vi "PID Advanced (DBL Array) Obsolete.vi"(0 "setpoint":dbl[](array[numeric])=[0.0] format="%.2f", 1 "output range":cluster{"output high":dbl, "output low":dbl}[](array[cluster])=[{"output high"=100.0, "output low"=-100.0}] {"output low" format="%.2f"; "output high" format="%.2f"}, 2 "auto? (T)":bool[](array[boolean])=[TRUE], 3 "manual control":dbl[](array[numeric])=[0.0] format="%.2f", 5 "process variable":dbl[](array[numeric])=[0.0] format="%.2f", 7 "setpoint range":T2(array[cluster])=[{"setpoint high"=100.0, "setpoint low"=0.0}] {"setpoint high" format="%.2f"; "setpoint low" format="%.2f"}, 9 "PID gains":T1(array[cluster])=[{"proportional gain (Kc)"=1.0, "integral time (Ti, min)"=0.01, "derivative time (Td, min)"=0.0}] {"derivative time (Td, min)" format="%.3f"; "integral time (Ti, min)" format="%.3f"; "proportional gain (Kc)" format="%.3f"}, 11 "dt (s)":dbl=-1.0 format="%.3f", 12 "reinitialize? (F)":bool, 13 "beta":dbl[](array[numeric])=[1.0] format="%.2f", 14 "linearity":dbl[](array[numeric])=[1.0] format="%.2f") -> (4 "output":dbl[](array[numeric]) format="%.2f", 15 "dt out (s)":dbl format="%.3f")   [LabVIEW 2017, in "NI_PID_pid.lvlib"]
doc: "PID algorithm with advanced optional features. PID algorithm includes features of PID.vi as well as manual mode control with bumpless manual to automatic transitions, non-linear integral action, two degree of freedom control and error-squared control."
uses:
  <vilib>/addons/control/pid/NI_PID_pid.lvlib
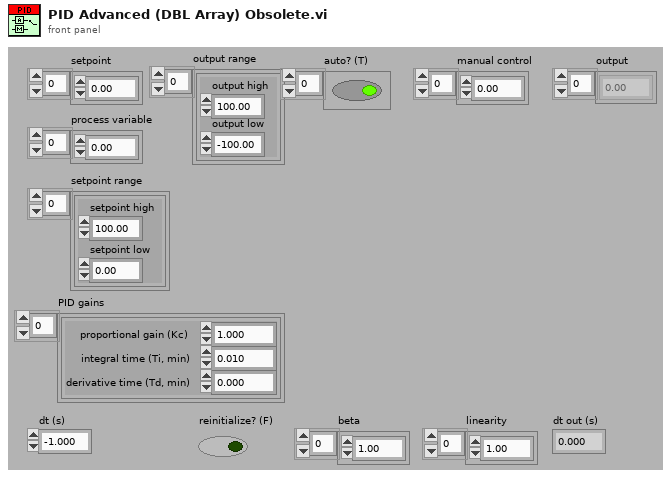
[diagram p1: front panel]
types:
  T1 = cluster{"proportional gain (Kc)":dbl, "integral time (Ti, min)":dbl, "derivative time (Td, min)":dbl}[]
  T2 = cluster{"setpoint high":dbl, "setpoint low":dbl}[]
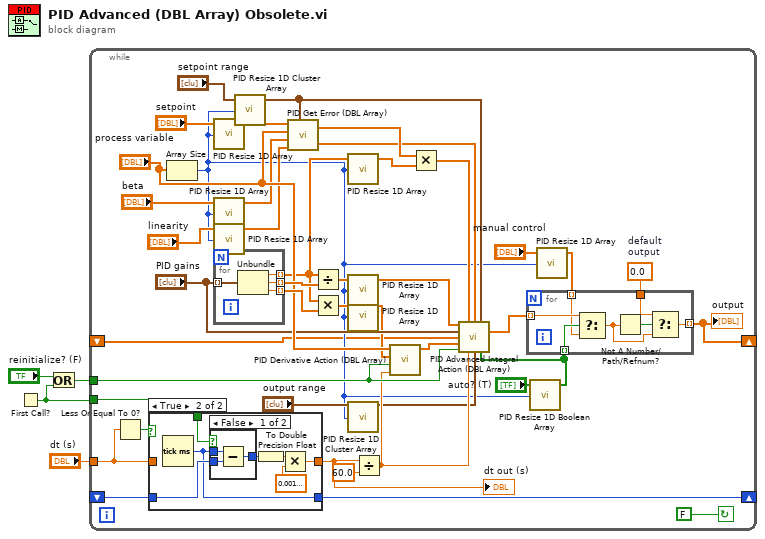
[diagram p0: block diagram]
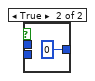
[diagram p3: hidden frame]
diagram:
  n1 = First Call?() -> (First Call?: T/F=w1:bool)
  n2 = Or(x="reinitialize? (F)", y=w1) -> (x .or. y?=w4:bool)
  n3 = while {
    shift-left: _ -> [w12]
    shift-right: [w13] -> _
    tunnel: w4 -> [w42]
    shift-left: _ -> [w6]
    shift-right: [w8] -> _
    tunnel: "dt (s)" -> [w9]
    tunnel: w1 -> [w5]
    stop <- FALSE continue-if-true
    w38 = 0.0  # default output
    n4 = Less Or Equal To 0?(x=w9) -> (x <= 0?=w10:bool)
    n5 = case shown="True" w10 {
      tunnel: [w49 w53] -> w7
      tunnel: w6 -> [w48 w52]
      tunnel: [w48 w51] -> w8
      tunnel: w9 -> [w49 _]
      tunnel: w5 -> [_ w50]
      frame False {
      }
      frame True {
        n6 = Tick Count (ms)() -> (millisecond timer value=w51:u32)
        n7 = case shown="False" w50 {
          tunnel: [w59 u32 0] -> w55
          tunnel: w52 -> [w58 _]
          tunnel: w51 -> [w57 _]
          frame False {
            n8 = Subtract(x=w57, y=w58) -> (x-y=w59:u32)
          }
          frame True {
          }
        }
        n9 = To Double Precision Float(number=w55) -> (double precision float=w54:dbl)
        n10 = Multiply(x=w54, y=0.0010000000474974513) -> (x*y=w53:dbl)
      }
    }
    "dt out (s)" <- w7
    n11 = Array Size(array="process variable") -> (size(s)=w15:i32)
    n12 = call <vilib>:"PID Resize 1D Array.vi"("array size"=w15, "input array"="setpoint") -> ("output array"=w35:dbl[])  [unwired: 3 out]
    n13 = call <vilib>:"PID Resize 1D Array.vi"("array size"=w15, "input array"="beta") -> ("output array"=w28:dbl[])  [unwired: 3 out]
    n14 = call <vilib>:"PID Resize 1D Array.vi"("array size"=w15, "input array"="linearity") -> ("output array"=w29:dbl[])  [unwired: 3 out]
    n15 = for {
      tunnel: [w71] -> w46 mode=indexing
      tunnel: [w70] -> w45 mode=indexing
      tunnel: [w69] -> w25 mode=indexing
      tunnel: "PID gains" -> [w68] mode=indexing
      n16 = Unbundle(w68) -> ("proportional gain (Kc)"=w69:dbl, "integral time (Ti, min)"=w71:dbl, "derivative time (Td, min)"=w70:dbl)
    }
    n17 = call <vilib>:"PID Resize 1D Cluster Array.vi"("array size"=w15, "input array"="setpoint range") -> ("output array"=w32:cluster{"output high":dbl, "output low":dbl}[])  [unwired: 3 out]
    n18 = call <vilib>:"PID Get Error (DBL Array).vi"("setpoint"=w35, "process variable"="process variable", "beta"=w28, "linearity"=w29, "setpoint range"=w32) -> ("error (with beta)"=w40:dbl[], "error"=w39:dbl[])
    n19 = Divide(x=w25, y=w46) -> (x/y=w21:dbl[])
    n20 = Multiply(x=w25, y=w45) -> (x*y=w24:dbl[])
    n21 = call <vilib>:"PID Resize 1D Array.vi"("array size"=w15, "input array"=w25) -> ("output array"=w26:dbl[])  [unwired: 3 out]
    n22 = call <vilib>:"PID Resize 1D Array.vi"("array size"=w15, "input array"=w21) -> ("output array"=w22:dbl[])  [unwired: 3 out]
    n23 = call <vilib>:"PID Resize 1D Array.vi"("array size"=w15, "input array"=w24) -> ("output array"=w23:dbl[])  [unwired: 3 out]
    n24 = call <vilib>:"PID Resize 1D Cluster Array.vi"("array size"=w15, "input array"="output range") -> ("output array"=w19:cluster{"output high":dbl, "output low":dbl}[])  [unwired: 3 out]
    n25 = Divide(x=w7, y=60.0) -> (x/y=w41:dbl)
    n26 = call <vilib>:"PID Derivative Action (DBL Array).vi"("dt (min)"=w41, "initialize (F)"=w42, "Kd"=w23, "process variable"="process variable") -> ("derivative action"=w43:dbl[])  [unwired: 3 out]
    n27 = Multiply(x=w40, y=w26) -> (x*y=w44:dbl[])
    n28 = call <vilib>:"PID Resize 1D Boolean Array.vi"("array size"=w15, "input array"="auto? (T)") -> ("output array"=w14:bool[])  [unwired: 3 out]
    n29 = call <vilib>:"PID Advanced Integral Action (DBL Array).vi"("Ki"=w22, "proportional action"=w44, "error"=w39, "setpoint range"=w32, "PID gains"="PID gains", "previous output"=w12, "derivative action"=w43, "initialize (F)"=w42, "dt (min)"=w41, "output range"=w19, "auto? (T)"=w14) -> ("output"=w37:dbl[])  [unwired: 4 out]
    n30 = call <vilib>:"PID Resize 1D Array.vi"("array size"=w15, "input array"="manual control") -> ("output array"=w17:dbl[])  [unwired: 3 out]
    n31 = for {
      tunnel: w38 -> [w67]
      tunnel: w37 -> [w65] mode=indexing
      tunnel: w14 -> [w63] mode=indexing
      tunnel: w17 -> [w62] mode=indexing
      tunnel: [w61] -> w13 mode=indexing
      n32 = Select(t=w65, s=w63, f=w62) -> (s? t:f=w64:dbl)
      n33 = Not A Number/Path/Refnum?(number/path/refnum=w64) -> (NaN/Path/Refnum?=w66:bool)
      n34 = Select(t=w67, s=w66, f=w64) -> (s? t:f=w61:dbl)
    }
    "output" <- w13
  }
